vi "current sweep mag sensor.vi"() -> ()   [LabVIEW 2012]
uses:
  <vilib>/DAQmx/write.llb/DAQmx Write (Analog 1D DBL 1Chan NSamp).vi
  <vilib>/DAQmx/read.llb/DAQmx Read (Analog 1D Wfm NChan NSamp).vi
  <vilib>/DAQmx/create/channels.llb/DAQmx Create Channel (AI-Voltage-Basic).vi
  <vilib>/DAQmx/create/channels.llb/DAQmx Create Channel (AO-Voltage-Basic).vi
  <vilib>/Analysis/1siggen.llb/Ramp Pattern by Samples.vi
  <vilib>/DAQmx/configure/timing.llb/DAQmx Timing (Sample Clock).vi
  <vilib>/DAQmx/miscellaneous.llb/DAQmx Fill In Error Info.vi
  <vilib>/Analysis/NI_AALBase.lvlib
panel:
  out "Waveform Graph":waveform(dbl)[](graph)
  in  "end":dbl=1.0 format="%0.2f"
  in  "start":dbl format="%0.2f"
  in  "samples per channel":i32=1000
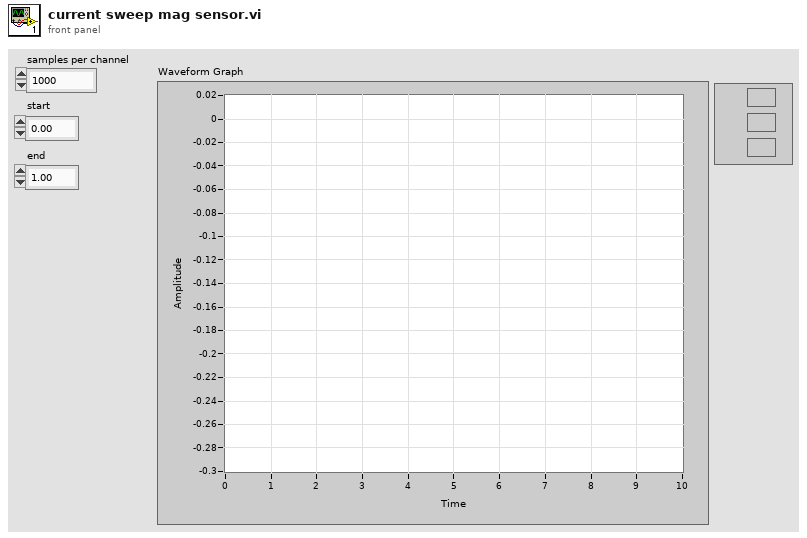
[diagram p1: front panel]
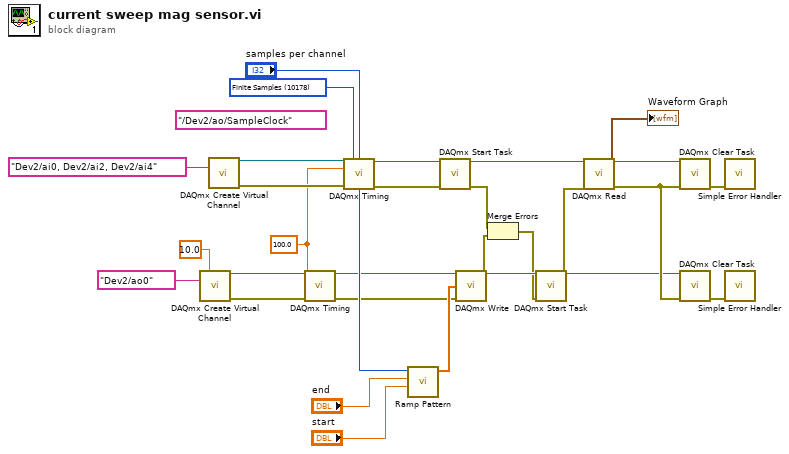
[diagram p0: block diagram]
diagram:
  w11 = 100.0 ("rate")
  w26 = 10178 items=["Finite Samples"=10178, "Continuous Samples"=10123, "Hardware Timed Single Point"=12522] ("sample mode")
  (unwired) tag "/Dev2/ao/SampleClock" ("source")
  n1 = call-poly <vilib>:"DAQmx Create Virtual Channel.vi"("maximum value"=10.0, "physical channels"=tag "Dev2/ao0") -> ("task out"=w22:refnum<k21>, "error out"=w4:errorcluster)  [unwired: 12 in]
  n2 = call-poly <vilib>:"DAQmx Create Virtual Channel.vi"("physical channels"=tag "Dev2/ai0, Dev2/ai2, Dev2/ai4") -> ("task out"=w28:refnum<k21>, "error out"=w27:errorcluster)  [unwired: 13 in]
  n3 = call-poly <vilib>:"DAQmx Timing.vi"("task/channels in"=w22, "rate"=w11, "error in"=w4) -> ("task out"=w10:refnum<k21>, "error out"=w9:errorcluster)  [unwired: 11 in]
  n4 = call-poly <vilib>:"DAQmx Timing.vi"("task/channels in"=w28, "sample mode"=w26, "samples per channel"="samples per channel", "rate"=w11, "error in"=w27) -> ("task out"=w25:refnum<k21>, "error out"=w24:errorcluster)  [unwired: 9 in]
  n5 = call-poly <vilib>:"Ramp Pattern.vi"("start"="start", "end"="end", "samples"="samples per channel") -> ("Ramp Pattern"=w16:dbl[])  [unwired: 7 in, 1 out]
  n6 = call <vilib>:"DAQmx Start Task.vi"("task/channels in"=w25, "error in"=w24) -> ("task out"=w20:refnum<k21>, "error out"=w7:errorcluster)  [unwired: 12 in]
  n7 = call-poly <vilib>:"DAQmx Write.vi"("task/channels in"=w10, "data"=w16, "error in"=w9) -> ("task out"=w8:refnum<k21>, "error out"=w6:errorcluster)  [unwired: 10 in, 1 out]
  n8 = Merge Errors(w7, w6) -> (w5:errorcluster)
  n9 = call <vilib>:"DAQmx Start Task.vi"("task/channels in"=w8, "error in"=w5) -> ("task out"=w1:refnum<k21>, "error out"=w3:errorcluster)  [unwired: 12 in]
  n10 = call-poly <vilib>:"DAQmx Read.vi"("task/channels in"=w20, "error in"=w3) -> ("task out"=w13:refnum<k21>, "data"=→"Waveform Graph":waveform(dbl)[], "error out"=w2:errorcluster)  [unwired: 11 in]
  n11 = call <vilib>:"DAQmx Clear Task.vi"("task in"=w13, "error in"=w2) -> ("error out"=w15:errorcluster)  [unwired: 13 in]
  n12 = call <vilib>:"DAQmx Clear Task.vi"("task in"=w1, "error in"=w2) -> ("error out"=w14:errorcluster)  [unwired: 13 in]
  n13 = call <vilib>:"Simple Error Handler.vi"("error in (no error)"=w15) -> ()  [unwired: 4 in, 5 out]
  n14 = call <vilib>:"Simple Error Handler.vi"("error in (no error)"=w14) -> ()  [unwired: 4 in, 5 out]
